vi "main.vi"() -> ()   [LabVIEW 2023] (continued)
  in  "Array":T2(array[cluster])=[{"1429FF9B", "Frame"="AirCompr1\ndatabase", "NameShort"="AirCompr1Curr", "StartBit"=32, "NumBits"=8, "Min"=0.0, "Max"=100.0, "ScaleFac"=1.0, "ScaleOff"=0.0}, {"1429FF9B", "Frame"="AirCompr1\ndatabase", "NameShort"="AirCompr1ErrCode", "StartBit"=56, "NumBits"=4, "Min"=0.0, "Max"=1.0, "ScaleFac"=1.0, "ScaleOff"=0.0}, {"1429FF9B", "Frame"="AirCompr1\ndatabase", "NameShort"="AirCompr1Life", "StartBit"=48, "NumBits"=8, "Min"=0.0, "Max"=255.0, "ScaleFac"=1.0, "ScaleOff"=0.0}, {"1429FF9B", "Frame"="AirCompr1\ndatabase", "NameShort"="AirCompr1MtrSpeed", "StartBit"=0, "NumBits"=16, "Min"=0.0, "Max"=5000.0, "ScaleFac"=0.125, "ScaleOff"=0.0}, {"1429FF9B", "Frame"="AirCompr1\ndatabase", "NameShort"="AirCompr1PrechgStat", "StartBit"=63, "NumBits"=1, "Min"=0.0, "Max"=1.0, "ScaleFac"=1.0, "ScaleOff"=0.0}, {"1429FF9B", "Frame"="AirCompr1\ndatabase", "NameShort"="AirCompr1Stat", "StartBit"=60, "NumBits"=2, "Min"=0.0, "Max"=1.0, "ScaleFac"=1.0, "ScaleOff"=0.0}, {"1429FF9B", "Frame"="AirCompr1\ndatabase", "NameShort"="AirCompr1Temp", "StartBit"=40, "NumBits"=8, "Min"=-40.0, "Max"=210.0, "ScaleFac"=1.0, "ScaleOff"=-40.0}, {"1429FF9B", "Frame"="AirCompr1\ndatabase", "NameShort"="AirCompr1Volt", "StartBit"=16, "NumBits"=16, "Min"=0.0, "Max"=1000.0, "ScaleFac"=0.1, "ScaleOff"=0.0}, {"18FFC09E", "Frame"="AirCon\ndatabase", "NameShort"="AirConCommWarn", "StartBit"=47, "NumBits"=1, "Min"=0.0, "Max"=1.0, "ScaleFac"=1.0, "ScaleOff"=0.0}, {"18FFC09E", "Frame"="AirCon\ndatabase", "NameShort"="AirConCooling1DefrostValidation", "StartBit"=17, "NumBits"=1, "Min"=0.0, "Max"=1.0, "ScaleFac"=1.0, "ScaleOff"=0.0}, {"18FFC09E", "Frame"="AirCon\ndatabase", "NameShort"="AirConCooling1Validation", "StartBit"=23, "NumBits"=1, "Min"=0.0, "Max"=1.0, "ScaleFac"=1.0, "ScaleOff"=0.0}, {"18FFC09E", "Frame"="AirCon\ndatabase", "NameShort"="AirConCooling2DefrostValidation", "StartBit"=20, "NumBits"=1, "Min"=0.0, "Max"=1.0, "ScaleFac"=1.0, "ScaleOff"=0.0}, {"18FFC09E", "Frame"="AirCon\ndatabase", "NameShort"="AirConCooling2Validation", "StartBit"=21, "NumBits"=1, "Min"=0.0, "Max"=1.0, "ScaleFac"=1.0, "ScaleOff"=0.0}, {"18FFC09E", "Frame"="AirCon\ndatabase", "NameShort"="AirConEvaporator1SnsrOpenCircuit", "StartBit"=2, "NumBits"=1, "Min"=0.0, "Max"=1.0, "ScaleFac"=1.0, "ScaleOff"=0.0}, {"18FFC09E", "Frame"="AirCon\ndatabase", "NameShort"="AirConEvaporator2SnsrOpenCircuit", "StartBit"=3, "NumBits"=1, "Min"=0.0, "Max"=1.0, "ScaleFac"=1.0, "ScaleOff"=0.0}, {"18FFC09E", "Frame"="AirCon\ndatabase", "NameShort"="AirConHeatValidation", "StartBit"=16, "NumBits"=1, "Min"=0.0, "Max"=1.0, "ScaleFac"=1.0, "ScaleOff"=0.0}, {"18FFC09E", "Frame"="AirCon\ndatabase", "NameShort"="AirConHighSpeed", "StartBit"=15, "NumBits"=1, "Min"=0.0, "Max"=1.0, "ScaleFac"=1.0, "ScaleOff"=0.0}, {"18FFC09E", "Frame"="AirCon\ndatabase", "NameShort"="AirConIndoorTemp", "StartBit"=24, "NumBits"=8, "Min"=-30.0, "Max"=97.0, "ScaleFac"=0.5, "ScaleOff"=-30.0}, {"18FFC09E", "Frame"="AirCon\ndatabase", "NameShort"="AirConInverterFailure", "StartBit"=6, "NumBits"=1, "Min"=0.0, "Max"=1.0, "ScaleFac"=1.0, "ScaleOff"=0.0}, {"18FFC09E", "Frame"="AirCon\ndatabase", "NameShort"="AirConLife", "StartBit"=56, "NumBits"=8, "Min"=0.0, "Max"=255.0, "ScaleFac"=1.0, "ScaleOff"=0.0}, {"18FFC09E", "Frame"="AirCon\ndatabase", "NameShort"="AirConLowSpeed", "StartBit"=13, "NumBits"=1, "Min"=0.0, "Max"=1.0, "ScaleFac"=1.0, "ScaleOff"=0.0}, {"18FFC09E", "Frame"="AirCon\ndatabase", "NameShort"="AirConMidSpeed", "StartBit"=14, "NumBits"=1, "Min"=0.0, "Max"=1.0, "ScaleFac"=1.0, "ScaleOff"=0.0}, {"18FFC09E", "Frame"="AirCon\ndatabase", "NameShort"="AirConOutTempSensorOpenCircuit", "StartBit"=1, "NumBits"=1, "Min"=0.0, "Max"=1.0, "ScaleFac"=1.0, "ScaleOff"=0.0}, {"18FFC09E", "Frame"="AirCon\ndatabase", "NameShort"="AirConOutdoorTemp", "StartBit"=32, "NumBits"=8, "Min"=-30.0, "Max"=97.0, "ScaleFac"=0.5, "ScaleOff"=-30.0}, {"18FFC09E", "Frame"="AirCon\ndatabase", "NameShort"="AirConPowSupplyOverVolt", "StartBit"=4, "NumBits"=1, "Min"=0.0, "Max"=1.0, "ScaleFac"=1.0, "ScaleOff"=0.0}, {"18FFC09E", "Frame"="AirCon\ndatabase", "NameShort"="AirConPowSupplyUnderVolt", "StartBit"=5, "NumBits"=1, "Min"=0.0, "Max"=1.0, "ScaleFac"=1.0, "ScaleOff"=0.0}, {"18FFC09E", "Frame"="AirCon\ndatabase", "NameShort"="AirConPressureFailure", "StartBit"=7, "NumBits"=1, "Min"=0.0, "Max"=1.0, "ScaleFac"=1.0, "ScaleOff"=0.0}, {"18FFC09E", "Frame"="AirCon\ndatabase", "NameShort"="AirConReqHV", "StartBit"=55, "NumBits"=1, "Min"=0.0, "Max"=1.0, "ScaleFac"=1.0, "ScaleOff"=0.0}, {"18FFC09E", "Frame"="AirCon\ndatabase", "NameShort"="AirConSterilizationValidation", "StartBit"=19, "NumBits"=1, "Min"=0.0, "Max"=1.0, "ScaleFac"=1.0, "ScaleOff"=0.0}, {"18FFC09E", "Frame"="AirCon\ndatabase", "NameShort"="AirConTempSensorOpenCircuit", "StartBit"=0, "NumBits"=1, "Min"=0.0, "Max"=1.0, "ScaleFac"=1.0, "ScaleOff"=0.0}, {"18FFC09E", "Frame"="AirCon\ndatabase", "NameShort"="AirConVentilatorValidation", "StartBit"=18, "NumBits"=1, "Min"=0.0, "Max"=1.0, "ScaleFac"=1.0, "ScaleOff"=0.0}, {"CFFE2A0", "Frame"="BCMData1\ndatabase", "NameShort"="BCMBatteryCoolantTemperature", "StartBit"=16, "NumBits"=8, "Min"=-40.0, "Max"=210.0, "ScaleFac"=1.0, "ScaleOff"=-40.0}, {"CFFE2A0", "Frame"="BCMData1\ndatabase", "NameShort"="BCMFrontAirReservoirPressure", "StartBit"=24, "NumBits"=8, "Min"=0.0, "Max"=2000.0, "ScaleFac"=8.0, "ScaleOff"=0.0}, {"CFFE2A0", "Frame"="BCMData1\ndatabase", "NameShort"="BCMLeadAcidBatteryVoltage", "StartBit"=0, "NumBits"=8, "Min"=0.0, "Max"=50.0, "ScaleFac"=0.2, "ScaleOff"=0.0}, {"CFFE2A0", "Frame"="BCMData1\ndatabase", "NameShort"="BCMMotorCoolantTemperature", "StartBit"=8, "NumBits"=8, "Min"=-40.0, "Max"=210.0, "ScaleFac"=1.0, "ScaleOff"=-40.0}, {"CFFE2A0", "Frame"="BCMData1\ndatabase", "NameShort"="BCMRearAirReservoirPressure", "StartBit"=32, "NumBits"=8, "Min"=0.0, "Max"=2000.0, "ScaleFac"=8.0, "ScaleOff"=0.0}, {"CFFE1A0", "Frame"="BCMIO1\ndatabase", "NameShort"="BCMABSActuation", "StartBit"=50, "NumBits"=2, "Min"=0.0, "Max"=3.0, "ScaleFac"=1.0, "ScaleOff"=0.0}, {"CFFE1A0", "Frame"="BCMIO1\ndatabase", "NameShort"="BCMAlcoholInterlock", "StartBit"=48, "NumBits"=2, "Min"=0.0, "Max"=3.0, "ScaleFac"=1.0, "ScaleOff"=0.0}, {"CFFE1A0", "Frame"="BCMIO1\ndatabase", "NameShort"="BCMAutoHeadLight", "StartBit"=60, "NumBits"=2, "Min"=0.0, "Max"=3.0, "ScaleFac"=1.0, "ScaleOff"=0.0}, {"CFFE1A0", "Frame"="BCMIO1\ndatabase", "NameShort"="BCMBrakePadWarning", "StartBit"=52, "NumBits"=2, "Min"=0.0, "Max"=3.0, "ScaleFac"=1.0, "ScaleOff"=0.0}, {"CFFE1A0", "Frame"="BCMIO1\ndatabase", "NameShort"="BCMBrakeRegeneration", "StartBit"=32, "NumBits"=2, "Min"=0.0, "Max"=3.0, "ScaleFac"=1.0, "ScaleOff"=0.0}, {"CFFE1A0", "Frame"="BCMIO1\ndatabase", "NameShort"="BCMCallHelp", "StartBit"=16, "NumBits"=2, "Min"=0.0, "Max"=3.0, "ScaleFac"=1.0, "ScaleOff"=0.0}, {"CFFE1A0", "Frame"="BCMIO1\ndatabase", "NameShort"="BCMDoorSwitchCoverEmergency", "StartBit"=26, "NumBits"=2, "Min"=0.0, "Max"=3.0, "ScaleFac"=1.0, "ScaleOff"=0.0}, {"CFFE1A0", "Frame"="BCMIO1\ndatabase", "NameShort"="BCMECASKneeling", "StartBit"=36, "NumBits"=2, "Min"=0.0, "Max"=3.0, "ScaleFac"=1.0, "ScaleOff"=0.0}, {"CFFE1A0", "Frame"="BCMIO1\ndatabase", "NameShort"="BCMECASWarning", "StartBit"=38, "NumBits"=2, "Min"=0.0, "Max"=3.0, "ScaleFac"=1.0, "ScaleOff"=0.0}, {"CFFE1A0", "Frame"="BCMIO1\ndatabase", "NameShort"="BCMEmergencyStop", "StartBit"=44, "NumBits"=2, "Min"=0.0, "Max"=3.0, "ScaleFac"=1.0, "ScaleOff"=0.0}, {"CFFE1A0", "Frame"="BCMIO1\ndatabase", "NameShort"="BCMEscapeDoorOpen", "StartBit"=56, "NumBits"=2, "Min"=0.0, "Max"=3.0, "ScaleFac"=1.0, "ScaleOff"=0.0}, {"CFFE1A0", "Frame"="BCMIO1\ndatabase", "NameShort"="BCMFootBrake", "StartBit"=54, "NumBits"=2, "Min"=0.0, "Max"=3.0, "ScaleFac"=1.0, "ScaleOff"=0.0}, {"CFFE1A0", "Frame"="BCMIO1\ndatabase", "NameShort"="BCMFrontDoor", "StartBit"=18, "NumBits"=2, "Min"=0.0, "Max"=3.0, "ScaleFac"=1.0, "ScaleOff"=0.0}, {"CFFE1A0", "Frame"="BCMIO1\ndatabase", "NameShort"="BCMFrontDoorEmergencyOpen", "StartBit"=22, "NumBits"=2, "Min"=0.0, "Max"=3.0, "ScaleFac"=1.0, "ScaleOff"=0.0}, {"CFFE1A0", "Frame"="BCMIO1\ndatabase", "NameShort"="BCMFrontFogLight", "StartBit"=12, "NumBits"=2, "Min"=0.0, "Max"=3.0, "ScaleFac"=1.0, "ScaleOff"=0.0}, {"CFFE1A0", "Frame"="BCMIO1\ndatabase", "NameShort"="BCMFrontWindowDefog", "StartBit"=28, "NumBits"=2, "Min"=0.0, "Max"=3.0, "ScaleFac"=1.0, "ScaleOff"=0.0}, {"CFFE1A0", "Frame"="BCMIO1\ndatabase", "NameShort"="BCMHandBrake", "StartBit"=34, "NumBits"=2, "Min"=0.0, "Max"=3.0, "ScaleFac"=1.0, "ScaleOff"=0.0}, {"CFFE1A0", "Frame"="BCMIO1\ndatabase", "NameShort"="BCMHazardLight", "StartBit"=10, "NumBits"=2, "Min"=0.0, "Max"=3.0, "ScaleFac"=1.0, "ScaleOff"=0.0}, {"CFFE1A0", "Frame"="BCMIO1\ndatabase", "NameShort"="BCMHighBeams", "StartBit"=6, "NumBits"=2, "Min"=0.0, "Max"=3.0, "ScaleFac"=1.0, "ScaleOff"=0.0}, {"CFFE1A0", "Frame"="BCMIO1\ndatabase", "NameShort"="BCMLowBeams", "StartBit"=4, "NumBits"=2, "Min"=0.0, "Max"=3.0, "ScaleFac"=1.0, "ScaleOff"=0.0}, {"CFFE1A0", "Frame"="BCMIO1\ndatabase", "NameShort"="BCMMiddleDoor", "StartBit"=20, "NumBits"=2, "Min"=0.0, "Max"=3.0, "ScaleFac"=1.0, "ScaleOff"=0.0}, {"CFFE1A0", "Frame"="BCMIO1\ndatabase", "NameShort"="BCMMiddleDoorEmergencyOpen", "StartBit"=24, "NumBits"=2, "Min"=0.0, "Max"=3.0, "ScaleFac"=1.0, "ScaleOff"=0.0}, {"CFFE1A0", "Frame"="BCMIO1\ndatabase", "NameShort"="BCMMirrorDefog", "StartBit"=30, "NumBits"=2, "Min"=0.0, "Max"=3.0, "ScaleFac"=1.0, "ScaleOff"=0.0}, {"CFFE1A0", "Frame"="BCMIO1\ndatabase", "NameShort"="BCMPositionLight", "StartBit"=8, "NumBits"=2, "Min"=0.0, "Max"=3.0, "ScaleFac"=1.0, "ScaleOff"=0.0}, {"CFFE1A0", "Frame"="BCMIO1\ndatabase", "NameShort"="BCMRampBoard", "StartBit"=46, "NumBits"=2, "Min"=0.0, "Max"=3.0, "ScaleFac"=1.0, "ScaleOff"=0.0}, {"CFFE1A0", "Frame"="BCMIO1\ndatabase", "NameShort"="BCMRearFogLight", "StartBit"=14, "NumBits"=2, "Min"=0.0, "Max"=3.0, "ScaleFac"=1.0, "ScaleOff"=0.0}, {"CFFE1A0", "Frame"="BCMIO1\ndatabase", "NameShort"="BCMRearHatchOpen", "StartBit"=42, "NumBits"=2, "Min"=0.0, "Max"=3.0, "ScaleFac"=1.0, "ScaleOff"=0.0}, {"CFFE1A0", "Frame"="BCMIO1\ndatabase", "NameShort"="BCMReversingLight", "StartBit"=62, "NumBits"=2, "Min"=0.0, "Max"=3.0, "ScaleFac"=1.0, "ScaleOff"=0.0}, {"CFFE1A0", "Frame"="BCMIO1\ndatabase", "NameShort"="BCMRunningLight", "StartBit"=58, "NumBits"=2, "Min"=0.0, "Max"=3.0, "ScaleFac"=1.0, "ScaleOff"=0.0}, {"CFFE1A0", "Frame"="BCMIO1\ndatabase", "NameShort"="BCMStopBell", "StartBit"=40, "NumBits"=2, "Min"=0.0, "Max"=3.0, "ScaleFac"=1.0, "ScaleOff"=0.0}, {"CFFE1A0", "Frame"="BCMIO1\ndatabase", "NameShort"="BCMTurnLeft", "StartBit"=0, "NumBits"=2, "Min"=0.0, "Max"=3.0, "ScaleFac"=1.0, "ScaleOff"=0.0}, {"CFFE1A0", "Frame"="BCMIO1\ndatabase", "NameShort"="BCMTurnRight", "StartBit"=2, "NumBits"=2, "Min"=0.0, "Max"=3.0, "ScaleFac"=1.0, "ScaleOff"=0.0}, {"CFFD1A0", "Frame"="BCMIO2\ndatabase", "NameShort"="BCMKeySwitchACC", "StartBit"=2, "NumBits"=2, "Min"=0.0, "Max"=3.0, "ScaleFac"=1.0, "ScaleOff"=0.0}, {"CFFD1A0", "Frame"="BCMIO2\ndatabase", "NameShort"="BCMKeySwitchON", "StartBit"=4, "NumBits"=2, "Min"=0.0, "Max"=3.0, "ScaleFac"=1.0, "ScaleOff"=0.0}, {"CFFD1A0", "Frame"="BCMIO2\ndatabase", "NameShort"="BCMRoofEscapeWindowOpen", "StartBit"=8, "NumBits"=2, "Min"=0.0, "Max"=3.0, "ScaleFac"=1.0, "ScaleOff"=0.0}, {"CFFD1A0", "Frame"="BCMIO2\ndatabase", "NameShort"="BCMSeatBelt", "StartBit"=0, "NumBits"=2, "Min"=0.0, "Max"=3.0, "ScaleFac"=1.0, "ScaleOff"=0.0}, {"CFFD1A0", "Frame"="BCMIO2\ndatabase", "NameShort"="BCMSideEscapeWindowOpen", "StartBit"=10, "NumBits"=2, "Min"=0.0, "Max"=3.0, "ScaleFac"=1.0, "ScaleOff"=0.0}, {"CFFD1A0", "Frame"="BCMIO2\ndatabase", "NameShort"="BCMSteerWheelDetect", "StartBit"=6, "NumBits"=2, "Min"=0.0, "Max"=3.0, "ScaleFac"=1.0, "ScaleOff"=0.0}, {"18F13DF3", "Frame"="BMS01StatNRelay\ndatabase", "NameShort"="BMS01AirComprNDCDCNEhpsRelayStat", "StartBit"=59, "NumBits"=1, "Min"=0.0, "Max"=1.0, "ScaleFac"=1.0, "ScaleOff"=0.0}, {"18F13DF3", "Frame"="BMS01StatNRelay\ndatabase", "NameShort"="BMS01AirConRelayStat", "StartBit"=60, "NumBits"=1, "Min"=0.0, "Max"=1.0, "ScaleFac"=1.0, "ScaleOff"=0.0}, {"18F13DF3", "Frame"="BMS01StatNRelay\ndatabase", "NameShort"="BMS01BMSErrLv", "StartBit"=48, "NumBits"=3, "Min"=0.0, "Max"=1.0, "ScaleFac"=1.0, "ScaleOff"=0.0}, {"18F13DF3", "Frame"="BMS01StatNRelay\ndatabase", "NameShort"="BMS01BMSHVEmergCutoff", "StartBit"=56, "NumBits"=1, "Min"=0.0, "Max"=1.0, "ScaleFac"=1.0, "ScaleOff"=0.0}, {"18F13DF3", "Frame"="BMS01StatNRelay\ndatabase", "NameShort"="BMS01BMSPowerOffRequest", "StartBit"=51, "NumBits"=2, "Min"=0.0, "Max"=3.0, "ScaleFac"=1.0, "ScaleOff"=0.0}, {"18F13DF3", "Frame"="BMS01StatNRelay\ndatabase", "NameShort"="BMS01BMSSOC", "StartBit"=32, "NumBits"=16, "Min"=0.0, "Max"=100.0, "ScaleFac"=0.4, "ScaleOff"=0.0}, {"18F13DF3", "Frame"="BMS01StatNRelay\ndatabase", "NameShort"="BMS01BMSStat", "StartBit"=53, "NumBits"=3, "Min"=0.0, "Max"=7.0, "ScaleFac"=1.0, "ScaleOff"=0.0}, {"18F13DF3", "Frame"="BMS01StatNRelay\ndatabase", "NameShort"="BMS01BattChgRelayStat", "StartBit"=62, "NumBits"=1, "Min"=0.0, "Max"=1.0, "ScaleFac"=1.0, "ScaleOff"=0.0}, {"18F13DF3", "Frame"="BMS01StatNRelay\ndatabase", "NameShort"="BMS01BattCurr", "StartBit"=16, "NumBits"=16, "Min"=-1000.0, "Max"=1000.0, "ScaleFac"=0.1, "ScaleOff"=-1000.0}, {"18F13DF3", "Frame"="BMS01StatNRelay\ndatabase", "NameShort"="BMS01BattMainRelayStat", "StartBit"=63, "NumBits"=1, "Min"=0.0, "Max"=1.0, "ScaleFac"=1.0, "ScaleOff"=0.0}, {"18F13DF3", "Frame"="BMS01StatNRelay\ndatabase", "NameShort"="BMS01BattVolt", "StartBit"=0, "NumBits"=16, "Min"=0.0, "Max"=1000.0, "ScaleFac"=0.1, "ScaleOff"=0.0}, {"18F13DF3", "Frame"="BMS01StatNRelay\ndatabase", "NameShort"="BMS01DefrostRelayStat", "StartBit"=61, "NumBits"=1, "Min"=0.0, "Max"=1.0, "ScaleFac"=1.0, "ScaleOff"=0.0}, {"18F13DF3", "Frame"="BMS01StatNRelay\ndatabase", "NameShort"="BMS01MtrRelayStat", "StartBit"=58, "NumBits"=1, "Min"=0.0, "Max"=1.0, "ScaleFac"=1.0, "ScaleOff"=0.0}, {"18F13DF3", "Frame"="BMS01StatNRelay\ndatabase", "NameShort"="BMS01PrechgRelayStat", "StartBit"=57, "NumBits"=1, "Min"=0.0, "Max"=1.0, "ScaleFac"=1.0, "ScaleOff"=0.0}, {"18F13EF3", "Frame"="BMS02VoltDiff\ndatabase", "NameShort"="BMS02BattCellMaxTemp", "StartBit"=32, "NumBits"=8, "Min"=-40.0, "Max"=210.0, "ScaleFac"=1.0, "ScaleOff"=-40.0}, {"18F13EF3", "Frame"="BMS02VoltDiff\ndatabase", "NameShort"="BMS02BattCellMaxVolt", "StartBit"=0, "NumBits"=16, "Min"=0.0, "Max"=655.35, "ScaleFac"=0.01, "ScaleOff"=0.0}, {"18F13EF3", "Frame"="BMS02VoltDiff\ndatabase", "NameShort"="BMS02BattCellMinTemp", "StartBit"=40, "NumBits"=8, "Min"=-40.0, "Max"=210.0, "ScaleFac"=1.0, "ScaleOff"=-40.0}, {"18F13EF3", "Frame"="BMS02VoltDiff\ndatabase", "NameShort"="BMS02BattCellMinVolt", "StartBit"=16, "NumBits"=16, "Min"=0.0, "Max"=655.35, "ScaleFac"=0.01, "ScaleOff"=0.0}, {"18F13EF3", "Frame"="BMS02VoltDiff\ndatabase", "NameShort"="BMS02BattNominalCapacitykWh", "StartBit"=48, "NumBits"=16, "Min"=0.0, "Max"=65535.0, "ScaleFac"=1.0, "ScaleOff"=0.0}, {"18F140F3", "Frame"="BMS04Curr\ndatabase", "NameShort"="BMS04BattMaxChgCurr", "StartBit"=0, "NumBits"=16, "Min"=-1000.0, "Max"=1000.0, "ScaleFac"=0.1, "ScaleOff"=-1000.0}, {"18F140F3", "Frame"="BMS04Curr\ndatabase", "NameShort"="BMS04BattMaxDischgCurr", "StartBit"=16, "NumBits"=16, "Min"=-1000.0, "Max"=1000.0, "ScaleFac"=0.1, "ScaleOff"=-1000.0}, {"18F140F3", "Frame"="BMS04Curr\ndatabase", "NameShort"="BMS04BattMinSOCAllowed", "StartBit"=48, "NumBits"=8, "Min"=0.0, "Max"=100.0, "ScaleFac"=0.4, "ScaleOff"=0.0}, {"18F140F3", "Frame"="BMS04Curr\ndatabase", "NameShort"="BMS04BattPackAllowedMaxTemp", "StartBit"=32, "NumBits"=8, "Min"=-40.0, "Max"=210.0, "ScaleFac"=1.0, "ScaleOff"=-40.0}, {"18F140F3", "Frame"="BMS04Curr\ndatabase", "NameShort"="BMS04BattPackAllowedMinTemp", "StartBit"=40, "NumBits"=8, "Min"=-40.0, "Max"=210.0, "ScaleFac"=1.0, "ScaleOff"=-40.0}, {"18F141F3", "Frame"="BMS05Error\ndatabase", "NameShort"="BMS05BalanceSysStat", "StartBit"=24, "NumBits"=1, "Min"=0.0, "Max"=1.0, "ScaleFac"=1.0, "ScaleOff"=0.0}, {"18F141F3", "Frame"="BMS05Error\ndatabase", "NameShort"="BMS05BattCellOvervoltWarn", "StartBit"=12, "NumBits"=1, "Min"=0.0, "Max"=1.0, "ScaleFac"=1.0, "ScaleOff"=0.0}, {"18F141F3", "Frame"="BMS05Error\ndatabase", "NameShort"="BMS05BattCellUndervoltWarn", "StartBit"=13, "NumBits"=1, "Min"=0.0, "Max"=1.0, "ScaleFac"=1.0, "ScaleOff"=0.0}, {"18F141F3", "Frame"="BMS05Error\ndatabase", "NameShort"="BMS05BattCellVoltDiffWarn", "StartBit"=14, "NumBits"=1, "Min"=0.0, "Max"=1.0, "ScaleFac"=1.0, "ScaleOff"=0.0}, {"18F141F3", "Frame"="BMS05Error\ndatabase", "NameShort"="BMS05BowTypeChgStat", "StartBit"=40, "NumBits"=3, "Min"=0.0, "Max"=1.0, "ScaleFac"=1.0, "ScaleOff"=0.0}, {"18F141F3", "Frame"="BMS05Error\ndatabase", "NameShort"="BMS05CANVer", "StartBit"=56, "NumBits"=8, "Min"=0.0, "Max"=2.55, "ScaleFac"=0.01, "ScaleOff"=0.0}, {"18F141F3", "Frame"="BMS05Error\ndatabase", "NameShort"="BMS05ChgStat", "StartBit"=25, "NumBits"=2, "Min"=0.0, "Max"=1.0, "ScaleFac"=1.0, "ScaleOff"=0.0}, {"18F141F3", "Frame"="BMS05Error\ndatabase", "NameShort"="BMS05ChgSysMismatchWarn", "StartBit"=20, "NumBits"=1, "Min"=0.0, "Max"=1.0, "ScaleFac"=1.0, "ScaleOff"=0.0}, {"18F141F3", "Frame"="BMS05Error\ndatabase", "NameShort"="BMS05ErrCode", "StartBit"=0, "NumBits"=8, "Min"=0.0, "Max"=255.0, "ScaleFac"=1.0, "ScaleOff"=0.0}, {"18F141F3", "Frame"="BMS05Error\ndatabase", "NameShort"="BMS05HVInterlockDisconnectWarn", "StartBit"=21, "NumBits"=1, "Min"=0.0, "Max"=1.0, "ScaleFac"=1.0, "ScaleOff"=0.0}, {"18F141F3", "Frame"="BMS05Error\ndatabase", "NameShort"="BMS05HighTempWarn", "StartBit"=9, "NumBits"=1, "Min"=0.0, "Max"=1.0, "ScaleFac"=1.0, "ScaleOff"=0.0}, {"18F141F3", "Frame"="BMS05Error\ndatabase", "NameShort"="BMS05InsulationWarn", "StartBit"=19, "NumBits"=1, "Min"=0.0, "Max"=1.0, "ScaleFac"=1.0, "ScaleOff"=0.0}, {"18F141F3", "Frame"="BMS05Error\ndatabase", "NameShort"="BMS05Life", "StartBit"=48, "NumBits"=8, "Min"=0.0, "Max"=255.0, "ScaleFac"=1.0, "ScaleOff"=0.0}, {"18F141F3", "Frame"="BMS05Error\ndatabase", "NameShort"="BMS05OverChgWarn", "StartBit"=15, "NumBits"=1, "Min"=0.0, "Max"=1.0, "ScaleFac"=1.0, "ScaleOff"=0.0}, {"18F141F3", "Frame"="BMS05Error\ndatabase", "NameShort"="BMS05OvervoltWarn", "StartBit"=10, "NumBits"=1, "Min"=0.0, "Max"=1.0, "ScaleFac"=1.0, "ScaleOff"=0.0}, {"18F141F3", "Frame"="BMS05Error\ndatabase", "NameShort"="BMS05PluginStat", "StartBit"=32, "NumBits"=8, "Min"=0.0, "Max"=255.0, "ScaleFac"=1.0, "ScaleOff"=0.0}, {"18F141F3", "Frame"="BMS05Error\ndatabase", "NameShort"="BMS05SOCRadicalChangeWarn", "StartBit"=18, "NumBits"=1, "Min"=0.0, "Max"=1.0, "ScaleFac"=1.0, "ScaleOff"=0.0}, {"18F141F3", "Frame"="BMS05Error\ndatabase", "NameShort"="BMS05SOCTooHighWarn", "StartBit"=17, "NumBits"=1, "Min"=0.0, "Max"=1.0, "ScaleFac"=1.0, "ScaleOff"=0.0}, {"18F141F3", "Frame"="BMS05Error\ndatabase", "NameShort"="BMS05SOCTooLowWarn", "StartBit"=16, "NumBits"=1, "Min"=0.0, "Max"=1.0, "ScaleFac"=1.0, "ScaleOff"=0.0}, {"18F141F3", "Frame"="BMS05Error\ndatabase", "NameShort"="BMS05TempAbove75Warn", "StartBit"=22, "NumBits"=1, "Min"=0.0, "Max"=1.0, "ScaleFac"=1.0, "ScaleOff"=0.0}, {"18F141F3", "Frame"="BMS05Error\ndatabase", "NameShort"="BMS05TempAbove75WarnBoxNum", "StartBit"=27, "NumBits"=5, "Min"=0.0, "Max"=1.0, "ScaleFac"=1.0, "ScaleOff"=0.0}, {"18F141F3", "Frame"="BMS05Error\ndatabase", "NameShort"="BMS05TempDiffAbove30Warn", "StartBit"=8, "NumBits"=1, "Min"=0.0, "Max"=1.0, "ScaleFac"=1.0, "ScaleOff"=0.0}, {"18F141F3", "Frame"="BMS05Error\ndatabase", "NameShort"="BMS05UndervoltWarn", "StartBit"=11, "NumBits"=1, "Min"=0.0, "Max"=1.0, "ScaleFac"=1.0, "ScaleOff"=0.0}, {"18F142F3", "Frame"="BMS06\ndatabase", "NameShort"="BMS06BattMinTempPoint1", "StartBit"=0, "NumBits"=8, "Min"=-40.0, "Max"=210.0, "ScaleFac"=1.0, "ScaleOff"=-40.0}, {"18F142F3", "Frame"="BMS06\ndatabase", "NameShort"="BMS06BattMinTempPoint1BoxNum", "StartBit"=8, "NumBits"=8, "Min"=0.0, "Max"=100.0, "ScaleFac"=1.0, "ScaleOff"=0.0}, {"18F142F3", "Frame"="BMS06\ndatabase", "NameShort"="BMS06BattMinTempPoint2", "StartBit"=16, "NumBits"=8, "Min"=-40.0, "Max"=210.0, "ScaleFac"=1.0, "ScaleOff"=-40.0}, {"18F142F3", "Frame"="BMS06\ndatabase", "NameShort"="BMS06BattMinTempPoint2BoxNum", "StartBit"=24, "NumBits"=8, "Min"=0.0, "Max"=100.0, "ScaleFac"=1.0, "ScaleOff"=0.0}, {"18F142F3", "Frame"="BMS06\ndatabase", "NameShort"="BMS06BattMinTempPoint3", "StartBit"=32, "NumBits"=8, "Min"=-40.0, "Max"=210.0, "ScaleFac"=1.0, "ScaleOff"=-40.0}, {"18F142F3", "Frame"="BMS06\ndatabase", "NameShort"="BMS06BattMinTempPoint3BoxNum", "StartBit"=40, "NumBits"=8, "Min"=0.0, "Max"=100.0, "ScaleFac"=1.0, "ScaleOff"=0.0}, {"18F142F3", "Frame"="BMS06\ndatabase", "NameShort"="BMS06BattMinTempPoint4", "StartBit"=48, "NumBits"=8, "Min"=-40.0, "Max"=210.0, "ScaleFac"=1.0, "ScaleOff"=-40.0}, {"18F142F3", "Frame"="BMS06\ndatabase", "NameShort"="BMS06BattMinTempPoint4BoxNum", "StartBit"=56, "NumBits"=8, "Min"=0.0, "Max"=100.0, "ScaleFac"=1.0, "ScaleOff"=0.0}, {"18F143F3", "Frame"="BMS07\ndatabase", "NameShort"="BMS06BattMaxTempPoint1", "StartBit"=0, "NumBits"=8, "Min"=-40.0, "Max"=210.0, "ScaleFac"=1.0, "ScaleOff"=-40.0}, {"18F143F3", "Frame"="BMS07\ndatabase", "NameShort"="BMS06BattMaxTempPoint1BoxNum", "StartBit"=8, "NumBits"=8, "Min"=0.0, "Max"=100.0, "ScaleFac"=1.0, "ScaleOff"=0.0}, {"18F143F3", "Frame"="BMS07\ndatabase", "NameShort"="BMS06BattMaxTempPoint2", "StartBit"=16, "NumBits"=8, "Min"=-40.0, "Max"=210.0, "ScaleFac"=1.0, "ScaleOff"=-40.0}, {"18F143F3", "Frame"="BMS07\ndatabase", "NameShort"="BMS06BattMaxTempPoint2BoxNum", "StartBit"=24, "NumBits"=8, "Min"=0.0, "Max"=100.0, "ScaleFac"=1.0, "ScaleOff"=0.0}, {"18F143F3", "Frame"="BMS07\ndatabase", "NameShort"="BMS06BattMaxTempPoint3", "StartBit"=32, "NumBits"=8, "Min"=-40.0, "Max"=210.0, "ScaleFac"=1.0, "ScaleOff"=-40.0}, {"18F143F3", "Frame"="BMS07\ndatabase", "NameShort"="BMS06BattMaxTempPoint3BoxNum", "StartBit"=40, "NumBits"=8, "Min"=0.0, "Max"=100.0, "ScaleFac"=1.0, "ScaleOff"=0.0}, {"18F143F3", "Frame"="BMS07\ndatabase", "NameShort"="BMS06BattMaxTempPoint4", "StartBit"=48, "NumBits"=8, "Min"=-40.0, "Max"=210.0, "ScaleFac"=1.0, "ScaleOff"=-40.0}, {"18F143F3", "Frame"="BMS07\ndatabase", "NameShort"="BMS06BattMaxTempPoint4BoxNum", "StartBit"=56, "NumBits"=8, "Min"=0.0, "Max"=100.0, "ScaleFac"=1.0, "ScaleOff"=0.0}, {"18F144F3", "Frame"="BMS08\ndatabase", "NameShort"="BMS08BattCellMinVolt1", "StartBit"=0, "NumBits"=16, "Min"=0.0, "Max"=655.35, "ScaleFac"=0.01, "ScaleOff"=0.0}, {"18F144F3", "Frame"="BMS08\ndatabase", "NameShort"="BMS08BattCellMinVolt1Box", "StartBit"=24, "NumBits"=8, "Min"=0.0, "Max"=255.0, "ScaleFac"=1.0, "ScaleOff"=0.0}, {"18F144F3", "Frame"="BMS08\ndatabase", "NameShort"="BMS08BattCellMinVolt1Num", "StartBit"=16, "NumBits"=8, "Min"=0.0, "Max"=100.0, "ScaleFac"=1.0, "ScaleOff"=0.0}, {"18F144F3", "Frame"="BMS08\ndatabase", "NameShort"="BMS08BattCellMinVolt2", "StartBit"=32, "NumBits"=16, "Min"=0.0, "Max"=655.35, "ScaleFac"=0.01, "ScaleOff"=0.0}, {"18F144F3", "Frame"="BMS08\ndatabase", "NameShort"="BMS08BattCellMinVolt2Box", "StartBit"=56, "NumBits"=8, "Min"=0.0, "Max"=255.0, "ScaleFac"=1.0, "ScaleOff"=0.0}, {"18F144F3", "Frame"="BMS08\ndatabase", "NameShort"="BMS08BattCellMinVolt2Num", "StartBit"=48, "NumBits"=8, "Min"=0.0, "Max"=100.0, "ScaleFac"=1.0, "ScaleOff"=0.0}, {"18F145F3", "Frame"="BMS09\ndatabase", "NameShort"="BMS09BattCellMinVolt3", "StartBit"=0, "NumBits"=16, "Min"=0.0, "Max"=655.35, "ScaleFac"=0.01, "ScaleOff"=0.0}, {"18F145F3", "Frame"="BMS09\ndatabase", "NameShort"="BMS09BattCellMinVolt3Box", "StartBit"=24, "NumBits"=8, "Min"=0.0, "Max"=255.0, "ScaleFac"=1.0, "ScaleOff"=0.0}, {"18F145F3", "Frame"="BMS09\ndatabase", "NameShort"="BMS09BattCellMinVolt3Num", "StartBit"=16, "NumBits"=8, "Min"=0.0, "Max"=100.0, "ScaleFac"=1.0, "ScaleOff"=0.0}, {"18F145F3", "Frame"="BMS09\ndatabase", "NameShort"="BMS09BattCellMinVolt4", "StartBit"=32, "NumBits"=16, "Min"=0.0, "Max"=655.35, "ScaleFac"=0.01, "ScaleOff"=0.0}, {"18F145F3", "Frame"="BMS09\ndatabase", "NameShort"="BMS09BattCellMinVolt4Box", "StartBit"=56, "NumBits"=8, "Min"=0.0, "Max"=255.0, "ScaleFac"=1.0, "ScaleOff"=0.0}, {"18F145F3", "Frame"="BMS09\ndatabase", "NameShort"="BMS09BattCellMinVolt4Num", "StartBit"=48, "NumBits"=8, "Min"=0.0, "Max"=100.0, "ScaleFac"=1.0, "ScaleOff"=0.0}, {"18F146F3", "Frame"="BMS10\ndatabase", "NameShort"="BMS10BattCellMinVolt1", "StartBit"=0, "NumBits"=16, "Min"=0.0, "Max"=655.35, "ScaleFac"=0.01, "ScaleOff"=0.0}, {"18F146F3", "Frame"="BMS10\ndatabase", "NameShort"="BMS10BattCellMinVolt1Box", "StartBit"=24, "NumBits"=8, "Min"=0.0, "Max"=255.0, "ScaleFac"=1.0, "ScaleOff"=0.0}, {"18F146F3", "Frame"="BMS10\ndatabase", "NameShort"="BMS10BattCellMinVolt1Num", "StartBit"=16, "NumBits"=8, "Min"=0.0, "Max"=100.0, "ScaleFac"=1.0, "ScaleOff"=0.0}, {"18F146F3", "Frame"="BMS10\ndatabase", "NameShort"="BMS10BattCellMinVolt2", "StartBit"=32, "NumBits"=16, "Min"=0.0, "Max"=655.35, "ScaleFac"=0.01, "ScaleOff"=0.0}, {"18F146F3", "Frame"="BMS10\ndatabase", "NameShort"="BMS10BattCellMinVolt2Box", "StartBit"=56, "NumBits"=8, "Min"=0.0, "Max"=255.0, "ScaleFac"=1.0, "ScaleOff"=0.0}, {"18F146F3", "Frame"="BMS10\ndatabase", "NameShort"="BMS10BattCellMinVolt2Num", "StartBit"=48, "NumBits"=8, "Min"=0.0, "Max"=100.0, "ScaleFac"=1.0, "ScaleOff"=0.0}, {"18F147F3", "Frame"="BMS11\ndatabase", "NameShort"="BMS11BattCellMinVolt3", "StartBit"=0, "NumBits"=16, "Min"=0.0, "Max"=655.35, "ScaleFac"=0.01, "ScaleOff"=0.0}, {"18F147F3", "Frame"="BMS11\ndatabase", "NameShort"="BMS11BattCellMinVolt3Box", "StartBit"=24, "NumBits"=8, "Min"=0.0, "Max"=255.0, "ScaleFac"=1.0, "ScaleOff"=0.0}, {"18F147F3", "Frame"="BMS11\ndatabase", "NameShort"="BMS11BattCellMinVolt3Num", "StartBit"=16, "NumBits"=8, "Min"=0.0, "Max"=100.0, "ScaleFac"=1.0, "ScaleOff"=0.0}, {"18F147F3", "Frame"="BMS11\ndatabase", "NameShort"="BMS11BattCellMinVolt4", "StartBit"=32, "NumBits"=16, "Min"=0.0, "Max"=655.35, "ScaleFac"=0.01, "ScaleOff"=0.0}, {"18F147F3", "Frame"="BMS11\ndatabase", "NameShort"="BMS11BattCellMinVolt4Box", "StartBit"=56, "NumBits"=8, "Min"=0.0, "Max"=255.0, "ScaleFac"=1.0, "ScaleOff"=0.0}, {"18F147F3", "Frame"="BMS11\ndatabase", "NameShort"="BMS11BattCellMinVolt4Num", "StartBit"=48, "NumBits"=8, "Min"=0.0, "Max"=100.0, "ScaleFac"=1.0, "ScaleOff"=0.0}, {"18F148F3", "Frame"="BMS12\ndatabase", "NameShort"="BMS12BattPackProdMonth", "StartBit"=40, "NumBits"=8, "Min"=0.0, "Max"=12.0, "ScaleFac"=1.0, "ScaleOff"=0.0}, {"18F148F3", "Frame"="BMS12\ndatabase", "NameShort"="BMS12BattPackProdYear", "StartBit"=32, "NumBits"=8, "Min"=1985.0, "Max"=2235.0, "ScaleFac"=1.0, "ScaleOff"=1985.0}, {"18F148F3", "Frame"="BMS12\ndatabase", "NameShort"="BMS12BattProdDay", "StartBit"=48, "NumBits"=8, "Min"=0.0, "Max"=31.0, "ScaleFac"=1.0, "ScaleOff"=0.0}, {"18F148F3", "Frame"="BMS12\ndatabase", "NameShort"="BMS12BattRatedCapacity", "StartBit"=0, "NumBits"=16, "Min"=0.0, "Max"=1000.0, "ScaleFac"=1.0, "ScaleOff"=0.0}, {"18F148F3", "Frame"="BMS12\ndatabase", "NameShort"="BMS12BattRatedVolt", "StartBit"=16, "NumBits"=16, "Min"=0.0, "Max"=1000.0, "ScaleFac"=1.0, "ScaleOff"=0.0}, {"18FFC3A9", "Frame"="BluestarAirConErrorNBoot\ndatabase", "NameShort"="BluestarAirConElectricBoxPow", "StartBit"=40, "NumBits"=2, "Min"=0.0, "Max"=2.0, "ScaleFac"=1.0, "ScaleOff"=0.0}, {"18FFC3A9", "Frame"="BluestarAirConErrorNBoot\ndatabase", "NameShort"="BluestarAirConErr01Overvoltage", "StartBit"=4, "NumBits"=2, "Min"=0.0, "Max"=1.0, "ScaleFac"=1.0, "ScaleOff"=0.0}, {"18FFC3A9", "Frame"="BluestarAirConErrorNBoot\ndatabase", "NameShort"="BluestarAirConErr02Undervoltage", "StartBit"=6, "NumBits"=2, "Min"=0.0, "Max"=1.0, "ScaleFac"=1.0, "ScaleOff"=0.0}, {"18FFC3A9", "Frame"="BluestarAirConErrorNBoot\ndatabase", "NameShort"="BluestarAirConErr03UnderPressure", "StartBit"=0, "NumBits"=2, "Min"=0.0, "Max"=2.0, "ScaleFac"=1.0, "ScaleOff"=0.0}, {"18FFC3A9", "Frame"="BluestarAirConErrorNBoot\ndatabase", "NameShort"="BluestarAirConErr04EDefroster", "StartBit"=14, "NumBits"=2, "Min"=0.0, "Max"=2.0, "ScaleFac"=1.0, "ScaleOff"=0.0}, {"18FFC3A9", "Frame"="BluestarAirConErrorNBoot\ndatabase", "NameShort"="BluestarAirConErr05IndoorSensor", "StartBit"=8, "NumBits"=2, "Min"=0.0, "Max"=2.0, "ScaleFac"=1.0, "ScaleOff"=0.0}, {"18FFC3A9", "Frame"="BluestarAirConErrorNBoot\ndatabase", "NameShort"="BluestarAirConErr07OverPressure", "StartBit"=2, "NumBits"=2, "Min"=0.0, "Max"=2.0, "ScaleFac"=1.0, "ScaleOff"=0.0}, {"18FFC3A9", "Frame"="BluestarAirConErrorNBoot\ndatabase", "NameShort"="BluestarAirConErr08OutdoorSensor", "StartBit"=10, "NumBits"=2, "Min"=0.0, "Max"=2.0, "ScaleFac"=1.0, "ScaleOff"=0.0}, {"18FFC3A9", "Frame"="BluestarAirConErrorNBoot\ndatabase", "NameShort"="BluestarAirConErr09Compressor", "StartBit"=32, "NumBits"=2, "Min"=0.0, "Max"=2.0, "ScaleFac"=1.0, "ScaleOff"=0.0}, {"18FFC3A9", "Frame"="BluestarAirConErrorNBoot\ndatabase", "NameShort"="BluestarAirConErr10Inverter", "StartBit"=28, "NumBits"=2, "Min"=0.0, "Max"=2.0, "ScaleFac"=1.0, "ScaleOff"=0.0}, {"18FFC2A9", "Frame"="BluestarAirConRemotePowerContro2\ndatabase", "NameShort"="BluestarAirConIndoorTemp", "StartBit"=0, "NumBits"=8, "Min"=-40.0, "Max"=210.0, "ScaleFac"=1.0, "ScaleOff"=-40.0}, {"18FFC2A9", "Frame"="BluestarAirConRemotePowerContro2\ndatabase", "NameShort"="BluestarAirConOutdoorTemp", "StartBit"=8, "NumBits"=8, "Min"=-40.0, "Max"=210.0, "ScaleFac"=1.0, "ScaleOff"=-40.0}, {"18FFC1A8", "Frame"="BluestarAirConRemotePowerControl\ndatabase", "NameShort"="BluestarAirConAutoMode", "StartBit"=44, "NumBits"=2, "Min"=0.0, "Max"=1.0, "ScaleFac"=1.0, "ScaleOff"=0.0}, {"18FFC1A8", "Frame"="BluestarAirConRemotePowerControl\ndatabase", "NameShort"="BluestarAirConFanSpeed", "StartBit"=4, "NumBits"=4, "Min"=0.0, "Max"=1.0, "ScaleFac"=1.0, "ScaleOff"=0.0}, {"18FFC1A8", "Frame"="BluestarAirConRemotePowerControl\ndatabase", "NameShort"="BluestarAirConMode", "StartBit"=8, "NumBits"=8, "Min"=0.0, "Max"=1.0, "ScaleFac"=1.0, "ScaleOff"=0.0}, {"18FFC1A8", "Frame"="BluestarAirConRemotePowerControl\ndatabase", "NameShort"="BluestarAirConPowerOnOff", "StartBit"=0, "NumBits"=2, "Min"=0.0, "Max"=1.0, "ScaleFac"=1.0, "ScaleOff"=0.0}, {"18FFC1A8", "Frame"="BluestarAirConRemotePowerControl\ndatabase", "NameShort"="BluestarAirConSetTemp", "StartBit"=16, "NumBits"=8, "Min"=-40.0, "Max"=210.0, "ScaleFac"=1.0, "ScaleOff"=-40.0}, {"142CFF98", "Frame"="DCDC\ndatabase", "NameShort"="DCDCErrCode", "StartBit"=56, "NumBits"=4, "Min"=0.0, "Max"=15.0, "ScaleFac"=1.0, "ScaleOff"=0.0}, {"142CFF98", "Frame"="DCDC\ndatabase", "NameShort"="DCDCINCurr", "StartBit"=16, "NumBits"=8, "Min"=0.0, "Max"=100.0, "ScaleFac"=1.0, "ScaleOff"=0.0}, {"142CFF98", "Frame"="DCDC\ndatabase", "NameShort"="DCDCINVolt", "StartBit"=0, "NumBits"=16, "Min"=0.0, "Max"=1000.0, "ScaleFac"=0.1, "ScaleOff"=0.0}, {"142CFF98", "Frame"="DCDC\ndatabase", "NameShort"="DCDCLife", "StartBit"=48, "NumBits"=8, "Min"=0.0, "Max"=255.0, "ScaleFac"=1.0, "ScaleOff"=0.0}, {"142CFF98", "Frame"="DCDC\ndatabase", "NameShort"="DCDCOUTCurr", "StartBit"=24, "NumBits"=8, "Min"=0.0, "Max"=100.0, "ScaleFac"=1.0, "ScaleOff"=0.0}, {"142CFF98", "Frame"="DCDC\ndatabase", "NameShort"="DCDCOUTVolt", "StartBit"=40, "NumBits"=8, "Min"=0.0, "Max"=100.0, "ScaleFac"=1.0, "ScaleOff"=0.0}, {"142CFF98", "Frame"="DCDC\ndatabase", "NameShort"="DCDCPrechgStat", "StartBit"=63, "NumBits"=1, "Min"=0.0, "Max"=1.0, "ScaleFac"=1.0, "ScaleOff"=0.0}, {"142CFF98", "Frame"="DCDC\ndatabase", "NameShort"="DCDCStat", "StartBit"=60, "NumBits"=2, "Min"=0.0, "Max"=1.0, "ScaleFac"=1.0, "ScaleOff"=0.0}, {"142CFF98", "Frame"="DCDC\ndatabase", "NameShort"="DCDCTemp", "StartBit"=32, "NumBits"=8, "Min"=-40.0, "Max"=200.0, "ScaleFac"=1.0, "ScaleOff"=-40.0}, {"142CFF97", "Frame"="DCDC2\ndatabase", "NameShort"="DCDC2ErrCode", "StartBit"=56, "NumBits"=4, "Min"=0.0, "Max"=15.0, "ScaleFac"=1.0, "ScaleOff"=0.0}, {"142CFF97", "Frame"="DCDC2\ndatabase", "NameShort"="DCDC2INCurr", "StartBit"=16, "NumBits"=8, "Min"=0.0, "Max"=100.0, "ScaleFac"=1.0, "ScaleOff"=0.0}, {"142CFF97", "Frame"="DCDC2\ndatabase", "NameShort"="DCDC2INVolt", "StartBit"=0, "NumBits"=16, "Min"=0.0, "Max"=1000.0, "ScaleFac"=0.1, "ScaleOff"=0.0}, {"142CFF97", "Frame"="DCDC2\ndatabase", "NameShort"="DCDC2Life", "StartBit"=48, "NumBits"=8, "Min"=0.0, "Max"=255.0, "ScaleFac"=1.0, "ScaleOff"=0.0}, {"142CFF97", "Frame"="DCDC2\ndatabase", "NameShort"="DCDC2OUTCurr", "StartBit"=24, "NumBits"=8, "Min"=0.0, "Max"=100.0, "ScaleFac"=1.0, "ScaleOff"=0.0}, {"142CFF97", "Frame"="DCDC2\ndatabase", "NameShort"="DCDC2OUTVolt", "StartBit"=40, "NumBits"=8, "Min"=0.0, "Max"=100.0, "ScaleFac"=1.0, "ScaleOff"=0.0}, {"142CFF97", "Frame"="DCDC2\ndatabase", "NameShort"="DCDC2PrechgStat", "StartBit"=63, "NumBits"=1, "Min"=0.0, "Max"=1.0, "ScaleFac"=1.0, "ScaleOff"=0.0}, {"142CFF97", "Frame"="DCDC2\ndatabase", "NameShort"="DCDC2Stat", "StartBit"=60, "NumBits"=2, "Min"=0.0, "Max"=1.0, "ScaleFac"=1.0, "ScaleOff"=0.0}, {"142CFF97", "Frame"="DCDC2\ndatabase", "NameShort"="DCDC2Temp", "StartBit"=32, "NumBits"=8, "Min"=-40.0, "Max"=200.0, "ScaleFac"=1.0, "ScaleOff"=-40.0}, {"142FFF95", "Frame"="Ehps1\ndatabase", "NameShort"="Ehps1Curr", "StartBit"=32, "NumBits"=8, "Min"=0.0, "Max"=100.0, "ScaleFac"=1.0, "ScaleOff"=0.0}, {"142FFF95", "Frame"="Ehps1\ndatabase", "NameShort"="Ehps1Life", "StartBit"=48, "NumBits"=8, "Min"=0.0, "Max"=255.0, "ScaleFac"=1.0, "ScaleOff"=0.0}, {"142FFF95", "Frame"="Ehps1\ndatabase", "NameShort"="Ehps1MalfuncCode1", "StartBit"=56, "NumBits"=4, "Min"=0.0, "Max"=15.0, "ScaleFac"=1.0, "ScaleOff"=0.0}, {"142FFF95", "Frame"="Ehps1\ndatabase", "NameShort"="Ehps1MtrSpeed", "StartBit"=0, "NumBits"=16, "Min"=0.0, "Max"=5000.0, "ScaleFac"=0.125, "ScaleOff"=0.0}, {"142FFF95", "Frame"="Ehps1\ndatabase", "NameShort"="Ehps1OilPumpStat", "StartBit"=60, "NumBits"=2, "Min"=0.0, "Max"=1.0, "ScaleFac"=1.0, "ScaleOff"=0.0}, {"142FFF95", "Frame"="Ehps1\ndatabase", "NameShort"="Ehps1PreChgStat", "StartBit"=63, "NumBits"=1, "Min"=0.0, "Max"=1.0, "ScaleFac"=1.0, "ScaleOff"=0.0}, {"142FFF95", "Frame"="Ehps1\ndatabase", "NameShort"="Ehps1Stat", "StartBit"=62, "NumBits"=1, "Min"=0.0, "Max"=1.0, "ScaleFac"=1.0, "ScaleOff"=0.0}, {"142FFF95", "Frame"="Ehps1\ndatabase", "NameShort"="Ehps1Temp", "StartBit"=40, "NumBits"=8, "Min"=-40.0, "Max"=210.0, "ScaleFac"=1.0, "ScaleOff"=-40.0}, {"142FFF95", "Frame"="Ehps1\ndatabase", "NameShort"="Ehps1Volt", "StartBit"=16, "NumBits"=16, "Min"=0.0, "Max"=1000.0, "ScaleFac"=0.1, "ScaleOff"=0.0}, {"18FFA7A9", "Frame"="FiveInOne\ndatabase", "NameShort"="FiveInOneAirComprRelayStat", "StartBit"=14, "NumBits"=2, "Min"=0.0, "Max"=1.0, "ScaleFac"=1.0, "ScaleOff"=0.0}, {"18FFA7A9", "Frame"="FiveInOne\ndatabase", "NameShort"="FiveInOneAirConRelayStat", "StartBit"=12, "NumBits"=2, "Min"=0.0, "Max"=1.0, "ScaleFac"=1.0, "ScaleOff"=0.0}, {"18FFA7A9", "Frame"="FiveInOne\ndatabase", "NameShort"="FiveInOneBrkResistRelayStat", "StartBit"=24, "NumBits"=2, "Min"=0.0, "Max"=1.0, "ScaleFac"=1.0, "ScaleOff"=0.0}, {"18FFA7A9", "Frame"="FiveInOne\ndatabase", "NameShort"="FiveInOneDCDCRelayStat", "StartBit"=2, "NumBits"=2, "Min"=0.0, "Max"=1.0, "ScaleFac"=1.0, "ScaleOff"=0.0}, {"18FFA7A9", "Frame"="FiveInOne\ndatabase", "NameShort"="FiveInOneDefrostRelayStat", "StartBit"=10, "NumBits"=2, "Min"=0.0, "Max"=1.0, "ScaleFac"=1.0, "ScaleOff"=0.0}, {"18FFA7A9", "Frame"="FiveInOne\ndatabase", "NameShort"="FiveInOneEHPSRelayStat", "StartBit"=0, "NumBits"=2, "Min"=0.0, "Max"=1.0, "ScaleFac"=1.0, "ScaleOff"=0.0}, {"18FFA7A9", "Frame"="FiveInOne\ndatabase", "NameShort"="FiveInOneHeaterRelayStat", "StartBit"=22, "NumBits"=2, "Min"=0.0, "Max"=1.0, "ScaleFac"=1.0, "ScaleOff"=0.0}, {"18FFA7A9", "Frame"="FiveInOne\ndatabase", "NameShort"="FiveInOneLife", "StartBit"=56, "NumBits"=8, "Min"=0.0, "Max"=255.0, "ScaleFac"=1.0, "ScaleOff"=0.0}, {"18FFA7A9", "Frame"="FiveInOne\ndatabase", "NameShort"="FiveInOneMtrRelayStat", "StartBit"=4, "NumBits"=2, "Min"=0.0, "Max"=1.0, "ScaleFac"=1.0, "ScaleOff"=0.0}, {"18FFA7A9", "Frame"="FiveInOne\ndatabase", "NameShort"="FiveInOnePluginStat", "StartBit"=8, "NumBits"=2, "Min"=0.0, "Max"=1.0, "ScaleFac"=1.0, "ScaleOff"=0.0}, {"18FFA7A9", "Frame"="FiveInOne\ndatabase", "NameShort"="FiveInOnePrechgRelayStat", "StartBit"=6, "NumBits"=2, "Min"=0.0, "Max"=1.0, "ScaleFac"=1.0, "ScaleOff"=0.0}, {"1801D0A7", "Frame"="INVTDCDCStat\ndatabase", "NameShort"="INVTDCDCFaultLvl", "StartBit"=8, "NumBits"=2, "Min"=0.0, "Max"=3.0, "ScaleFac"=1.0, "ScaleOff"=0.0}, {"1801D0A7", "Frame"="INVTDCDCStat\ndatabase", "NameShort"="INVTDCDCStatErrCode", "StartBit"=0, "NumBits"=8, "Min"=0.0, "Max"=255.0, "ScaleFac"=1.0, "ScaleOff"=0.0}, {"1801D0A7", "Frame"="INVTDCDCStat\ndatabase", "NameShort"="INVTDCDCStatFaultStat", "StartBit"=14, "NumBits"=2, "Min"=0.0, "Max"=3.0, "ScaleFac"=1.0, "ScaleOff"=0.0}, {"1801D0A7", "Frame"="INVTDCDCStat\ndatabase", "NameShort"="INVTDCDCStatINCurr", "StartBit"=32, "NumBits"=16, "Min"=0.0, "Max"=6553.5, "ScaleFac"=0.1, "ScaleOff"=0.0}, {"1801D0A7", "Frame"="INVTDCDCStat\ndatabase", "NameShort"="INVTDCDCStatINVolt", "StartBit"=16, "NumBits"=16, "Min"=0.0, "Max"=1000.0, "ScaleFac"=0.1, "ScaleOff"=0.0}, {"1801D0A7", "Frame"="INVTDCDCStat\ndatabase", "NameShort"="INVTDCDCStatLife", "StartBit"=56, "NumBits"=8, "Min"=0.0, "Max"=255.0, "ScaleFac"=1.0, "ScaleOff"=0.0}, {"1801D0A7", "Frame"="INVTDCDCStat\ndatabase", "NameShort"="INVTDCDCStatPowerStat", "StartBit"=10, "NumBits"=2, "Min"=0.0, "Max"=3.0, "ScaleFac"=1.0, "ScaleOff"=0.0}, {"1801D0A7", "Frame"="INVTDCDCStat\ndatabase", "NameShort"="INVTDCDCStatTemp", "StartBit"=48, "NumBits"=8, "Min"=-40.0, "Max"=200.0, "ScaleFac"=1.0, "ScaleOff"=-40.0}, {"1801D0A7", "Frame"="INVTDCDCStat\ndatabase", "NameShort"="INVTDCDCStatWorkStat", "StartBit"=12, "NumBits"=2, "Min"=0.0, "Max"=3.0, "ScaleFac"=1.0, "ScaleOff"=0.0}, {"1802D0A7", "Frame"="INVTDCDCStat2\ndatabase", "NameShort"="INVTDCDCStat2OUTCurr", "StartBit"=16, "NumBits"=16, "Min"=0.0, "Max"=500.0, "ScaleFac"=0.1, "ScaleOff"=0.0}, {"1802D0A7", "Frame"="INVTDCDCStat2\ndatabase", "NameShort"="INVTDCDCStat2OUTVolt", "StartBit"=0, "NumBits"=16, "Min"=0.0, "Max"=1000.0, "ScaleFac"=0.1, "ScaleOff"=0.0}, {"1801D0A6", "Frame"="INVTEACStat\ndatabase", "NameShort"="INVTEACFaultLvl", "StartBit"=8, "NumBits"=2, "Min"=0.0, "Max"=3.0, "ScaleFac"=1.0, "ScaleOff"=0.0}, {"1801D0A6", "Frame"="INVTEACStat\ndatabase", "NameShort"="INVTEACStatErrCode", "StartBit"=0, "NumBits"=8, "Min"=0.0, "Max"=255.0, "ScaleFac"=1.0, "ScaleOff"=0.0}, {"1801D0A6", "Frame"="INVTEACStat\ndatabase", "NameShort"="INVTEACStatFaultStat", "StartBit"=14, "NumBits"=2, "Min"=0.0, "Max"=3.0, "ScaleFac"=1.0, "ScaleOff"=0.0}, {"1801D0A6", "Frame"="INVTEACStat\ndatabase", "NameShort"="INVTEACStatINVolt", "StartBit"=16, "NumBits"=16, "Min"=0.0, "Max"=1000.0, "ScaleFac"=0.1, "ScaleOff"=0.0}, {"1801D0A6", "Frame"="INVTEACStat\ndatabase", "NameShort"="INVTEACStatInvertorTemp", "StartBit"=48, "NumBits"=8, "Min"=-40.0, "Max"=150.0, "ScaleFac"=1.0, "ScaleOff"=-40.0}, {"1801D0A6", "Frame"="INVTEACStat\ndatabase", "NameShort"="INVTEACStatLife", "StartBit"=56, "NumBits"=8, "Min"=0.0, "Max"=255.0, "ScaleFac"=1.0, "ScaleOff"=0.0}, {"1801D0A6", "Frame"="INVTEACStat\ndatabase", "NameShort"="INVTEACStatMtrTemp", "StartBit"=32, "NumBits"=8, "Min"=-40.0, "Max"=200.0, "ScaleFac"=1.0, "ScaleOff"=-40.0}, {"1801D0A6", "Frame"="INVTEACStat\ndatabase", "NameShort"="INVTEACStatPowerStat", "StartBit"=10, "NumBits"=2, "Min"=0.0, "Max"=3.0, "ScaleFac"=1.0, "ScaleOff"=0.0}, {"1801D0A6", "Frame"="INVTEACStat\ndatabase", "NameShort"="INVTEACStatWorkStat", "StartBit"=12, "NumBits"=2, "Min"=0.0, "Max"=3.0, "ScaleFac"=1.0, "ScaleOff"=0.0}, {"1802D0A6", "Frame"="INVTEACStat2\ndatabase", "NameShort"="INVTEACStat2INCurr", "StartBit"=48, "NumBits"=16, "Min"=0.0, "Max"=6553.5, "ScaleFac"=0.1, "ScaleOff"=0.0}, {"1802D0A6", "Frame"="INVTEACStat2\ndatabase", "NameShort"="INVTEACStat2Mtrrpm", "StartBit"=0, "NumBits"=16, "Min"=-5000.0, "Max"=5000.0, "ScaleFac"=0.5, "ScaleOff"=-5000.0}, {"1802D0A6", "Frame"="INVTEACStat2\ndatabase", "NameShort"="INVTEACStat2OUTCurr", "StartBit"=32, "NumBits"=16, "Min"=0.0, "Max"=500.0, 
